vi "DN4_Counter_SetPulseWidth_Ex.vi"(4 "error in (no error)":errorcluster, 5 "low period":dbl[](array[numeric]), 6 "high period":dbl[](array[numeric]), 7 "Task ID":u32) -> (0 "error out":errorcluster, 3 "Task ID":u32)   [LabVIEW 2009]
uses:
  Windows/System32/AdvLvDaq.dll
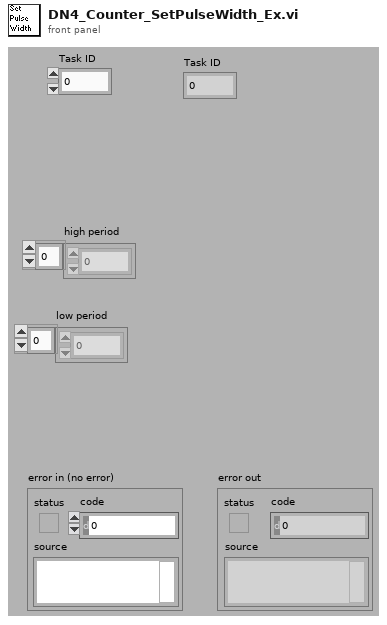
[diagram p1: front panel]
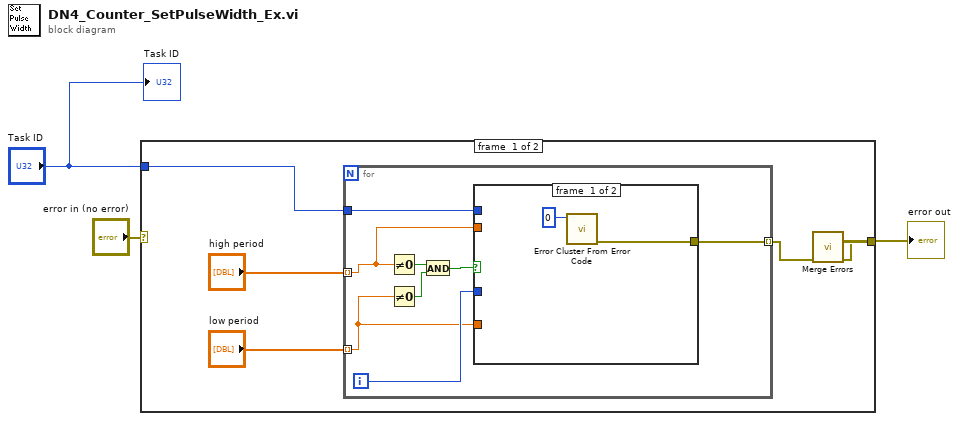
[diagram p0: block diagram]
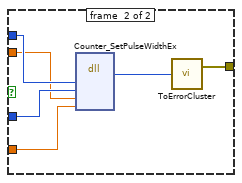
[diagram p2: hidden frame]
diagram:
  n1 = case shown="Error" "error in (no error)" {
    selector: "error in (no error)" -> [_ w25]
    tunnel: "Task ID" -> [w8 _]
    tunnel: [w7 w25] -> w2
    frame #0 {
      n2 = for {
        tunnel: [w13] -> w6 mode=indexing
        tunnel: w8 -> [w12]
        tunnel: "low period" -> [w9] mode=indexing
        tunnel: "high period" -> [w10] mode=indexing
        i -> [w11]
        n3 = Not Equal To 0?(x=w10) -> (x != 0?=w16:bool)
        n4 = Not Equal To 0?(x=w9) -> (x != 0?=w15:bool)
        n5 = And(x=w16, y=w15) -> (x .and. y?=w14:bool)
        n6 = case shown="True" w14 {
          tunnel: w12 -> [_ w24]
          tunnel: [w18 w23] -> w13
          tunnel: w11 -> [_ w21]
          tunnel: w10 -> [_ w20]
          tunnel: w9 -> [_ w19]
          frame #0 {
            n7 = call <vilib>:"Error Cluster From Error Code.vi"("error code (0)"=0) -> ("error out"=w18:errorcluster)  [unwired: 2 in, 6 out]
          }
          frame #1 {
            n8 = dll-call lib="C:/Windows/System32/AdvLvDaq.dll" fn="Counter_SetPulseWidthEx"("taskId"=w24, "channelIndex"=w21, "hiPeriod"=w20, "loPeriod"=w19) -> ("return type"=w22:i32)  [unwired: 7 in, 2 out]
            n9 = call <userlib>:"ToErrorCluster.vi"("error code"=w22) -> ("error out"=w23:errorcluster)
          }
        }
      }
      n10 = call <vilib>:"Merge Errors.vi"("error array in"=w6) -> ("error out"=w7:errorcluster)  [unwired: 3 in, 3 out]
    }
    frame #1 {
    }
  }
  "error out" <- w2
  "Task ID" <- "Task ID"
